vi "Start.vi"(11 "Plugin in":refnum<class "Plugin.lvclass">) -> (0 "error out":errorcluster, 3 "Plugin out":refnum<class "Plugin.lvclass">)   [LabVIEW 2024, in "FPGA Addon Engine.lvlib" / "Plugin.lvclass"]
uses:
  Plugin.lvclass
  Plugin.lvclass/Plugin.ctl
  <vilib>/rvi/interface/nirviMethod/nirviMethod.xnode
  <vilib>/rvi/interface/nirviMethod/StockFPGA_InlinedMethodWaitForSingleIRQ.vi
  <vilib>/FPGAPlugInAG/Dynamic/niLvFpga_WaitOnIrq_Dynamic.vi
  <vilib>/FPGAPlugInAG/Dynamic/niLvFpga_AcknowledgeIrq_Dynamic.vi
  VS Plugin Inline Async API/VS Plugin Inline Async API.lvclass
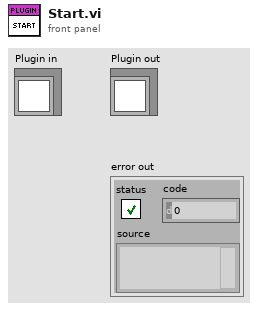
[diagram p1: front panel]
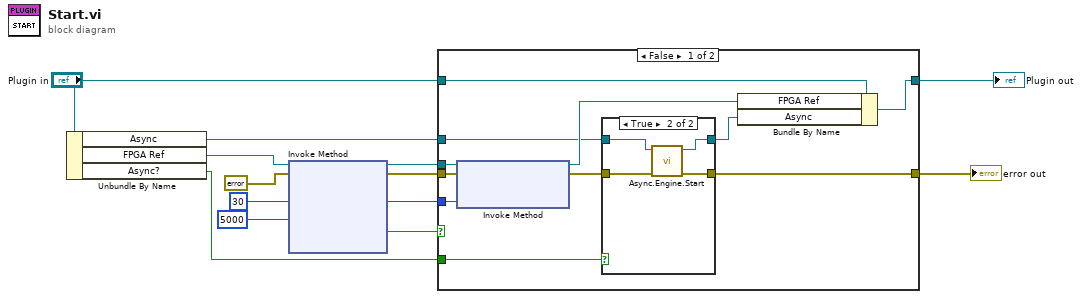
[diagram p0: block diagram]
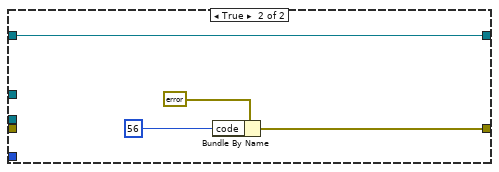
[diagram p3: hidden frame]
diagram:
  w7 = 30 ("IRQ Number(s)")
  n1 = Unbundle By Name("Plugin in") -> ("Async"=w3:refnum<class "VS Plugin Inline Async API.lvclass">, "FPGA Ref"=w9:refnum<k20>, "Async?"=w5:bool)
  n2 = xnode "Invoke Method"("FPGA VI Reference In"=w9, "error in"=errorcluster {"status"=FALSE, "code"=0, "source"=""}, "IRQ Number(s)"=w7, "Timeout (ms)"=5000) -> ("FPGA VI Reference Out"=w8:refnum<k20>, "error out"=w12:errorcluster, "Timed Out"=w4:bool)  [unwired: 1 out]
  n3 = case shown="False" w4 {
    tunnel: "Plugin in" -> [w14 w31]
    tunnel: [w13 w31] -> w2
    tunnel: w8 -> [w20 _]
    tunnel: w12 -> [w23 _]
    tunnel: w7 -> [w19 _]
    tunnel: w5 -> [w17 _]
    tunnel: w3 -> [w16 _]
    tunnel: [w21 w32] -> w10
    frame False {
      n4 = xnode "Invoke Method"("FPGA VI Reference In"=w20, "error in"=w23, "IRQ Number(s)"=w19) -> ("FPGA VI Reference Out"=w18:refnum<k20>, "error out"=w22:errorcluster)
      n5 = case shown="True" w17 {
        tunnel: w22 -> [w25 w29]
        tunnel: [w25 w28] -> w21
        tunnel: w16 -> [w24 w27]
        tunnel: [w24 w26] -> w15
        frame False {
        }
        frame True {
          n6 = call "Async.Engine.Start.vi"("error in"=w29, "VS Plugin Inline Async API in"=w27) -> ("error out"=w28:errorcluster, "VS Plugin Inline Async API out"=w26:refnum<class "VS Plugin Inline Async API.lvclass">)  [unwired: 8 in]
        }
      }
      n7 = Bundle By Name(cluster=w14, "FPGA Ref"=w18, "Async"=w15) -> (w13:refnum<class "Plugin.lvclass">)
    }
    frame True {
      n8 = Bundle By Name(cluster=errorcluster {"status"=FALSE, "code"=0, "source"=""} ("error in"), "code"=56) -> (w32:errorcluster)
    }
  }
  "error out" <- w10
  "Plugin out" <- w2
